vi "StartTest.vi"(8 "error in":errorcluster, 11 "TestInfo":T1) -> (0 "error out":errorcluster)   [LabVIEW 2018, in "S2.lvclass"]
uses:
  S2.lvclass
  Controller/Public Controls/TestInfo.ctl
  Queue/Queue Data.ctl
  Queue/State.ctl
  Controller/GUI.lvclass
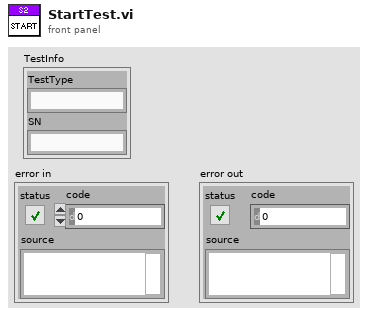
[diagram p1: front panel]
types:
  T1 = typedef "GUI.lvclass/TestInfo.ctl" = cluster{"TestType":string, "SN":string}
  T2 = typedef "S2.lvclass/Queue Data.ctl" = cluster{"State":T3, "Data":variant}
  T3 = typedef "S2.lvclass/State.ctl" = enum16{"Initialize", "SetConfig", "AckAlarm", "Alarm", "Idle", "LockLid", "LowPressure", "Pressurize", "DecayTest", "Vent", "Abort", "Start", "CreateReports", "WriteToReport", "WritePressure", "Error", "Exit"}
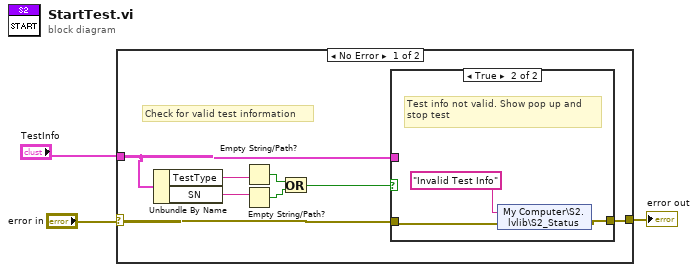
[diagram p0: block diagram]
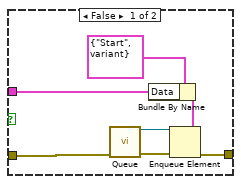
[diagram p2: hidden frame]
diagram:
  n1 = case shown="No Error" "error in" {
    selector: "error in" -> [w11 w22]
    tunnel: [w10 w22] -> w3
    tunnel: "TestInfo" -> [w9 _]
    frame No Error {
      # "Check for valid test information"
      n2 = Unbundle By Name(w9) -> ("TestType"=w7:string, "SN"=w8:string)
      n3 = Empty String/Path?(string/path=w7) -> (empty?=w6:bool)
      n4 = Empty String/Path?(string/path=w8) -> (empty?=w5:bool)
      n5 = Or(x=w6, y=w5) -> (x .or. y?=w4:bool)
      n6 = case shown="True" w4 {
        tunnel: w11 -> [w18 w20]
        tunnel: [w17 w19] -> w10
        tunnel: w9 -> [w14 _]
        frame False {
          n7 = call "Queue.vi"("error in"=w18) -> ("error out"=w12:errorcluster, "queue out"=w13:refnum<queue>)  [unwired: 9 in]
          n8 = Bundle By Name(cluster=T2 {"State"=enum."Start", "Data"=variant} ("element"), "Data"=w14) -> (w15:T2)
          n9 = Enqueue Element(queue=w13, element=w15, error in (no error)=w12) -> (error out=w17:errorcluster)  [unwired: 1 in, 2 out]
        }
        frame True {
          # "Test info not valid. Show pop up and\nstop test"
          n10 = shared-variable "My Computer\\S2.lvlib\\S2_Status"("Invalid Test Info" ("message"), error in=w20) -> (error out=w19:errorcluster)
        }
      }
    }
    frame Error {
    }
  }
  "error out" <- w3
